vi "单路通断器DEMO（半波整流）.vi"() -> ()   [LabVIEW 2012]
uses:
  <vilib>/Analysis/NI_AALBase.lvlib
panel:
  out "半波整流":dbl[](graph)
  out "半波整流":dbl[](graph)
  out "正弦波":dbl[](graph)
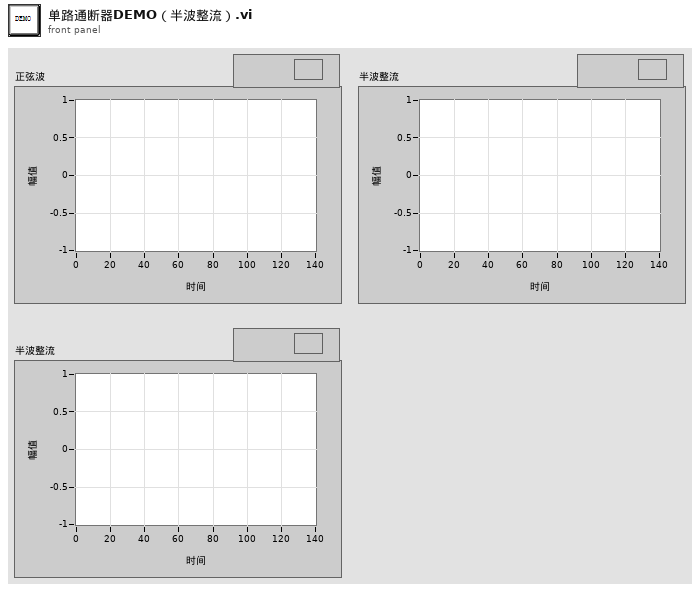
[diagram p1: front panel]
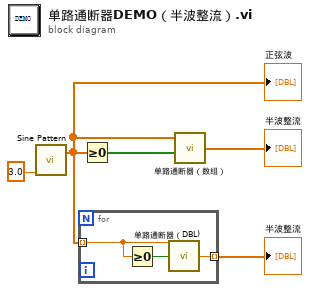
[diagram p0: block diagram]
diagram:
  n1 = call <vilib>:"Sine Pattern.vi"("cycles"=3.0) -> ("Sinusoidal Pattern"=w3:dbl[])  [unwired: 3 in, 1 out]
  "正弦波" <- w3
  n2 = for {
    tunnel: w3 -> [w8] mode=indexing
    tunnel: [w6] -> w4 mode=indexing
    n3 = Greater Or Equal To 0?(x=w8) -> (x >= 0?=w7:bool)
    n4 = call "单路通断器（DBL).vi"("直通？"=w7, "X_In"=w8) -> ("X_Out"=w6:dbl)  [unwired: 1 in]
  }
  "半波整流" <- w4
  n5 = Greater Or Equal To 0?(x=w3) -> (x >= 0?=w2:bool[])
  n6 = call-poly "单路通断器（数组）.vi"("直通？"=w2, "X_In"=w3) -> ("X_Out"=→"半波整流":dbl[])  [unwired: 1 in]
